vi "Table Select Section Cut to 1D Array.vi"(11 "Table Ref In":refnum<vi>) -> (1 "Cut Value":string[](array[string]), 3 "Table Ref Out":refnum<vi>)   [LabVIEW 2024]
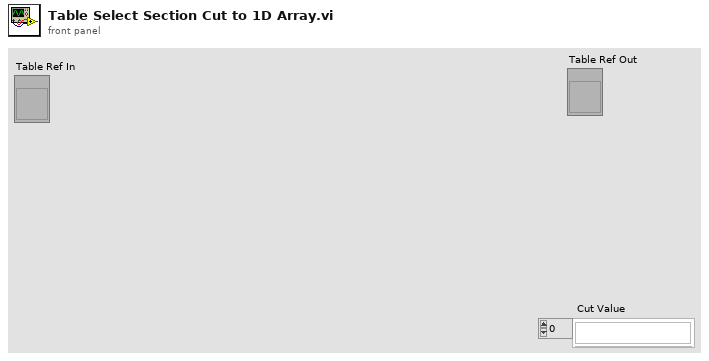
[diagram p1: front panel]
types:
  T1 = typedef "LVRowAndColumnTypeDef.ctl" = cluster{"Row":i32, "Column":i32}
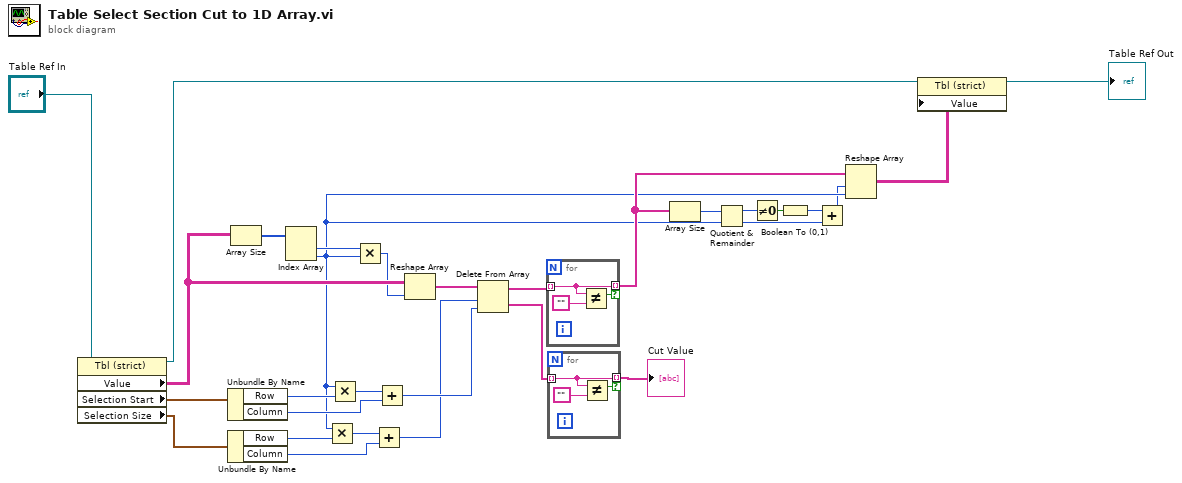
[diagram p0: block diagram]
diagram:
  n1 = property class="Tbl (strict)"(reference="Table Ref In") -> (reference out=w11:refnum<vi>, "Value"=w25:string[][], "Selection Start"=w29:T1, "Selection Size"=w28:T1)  [unwired: 1 in, 1 out]
  n2 = Unbundle By Name(w29) -> ("Row"=w23:i32, "Column"=w21:i32)
  n3 = Unbundle By Name(w28) -> ("Row"=w17:i32, "Column"=w16:i32)
  n4 = Array Size(array=w25) -> (size(s)=w27:i32[])
  n5 = Index Array(array=w27) -> (element #1=w26:i32, element #2=w7:i32)  [unwired: 2 in]
  n6 = Multiply(x=w7, y=w17) -> (x*y=w18:i32)
  n7 = Multiply(x=w7, y=w23) -> (x*y=w22:i32)
  n8 = Multiply(x=w26, y=w7) -> (x*y=w24:i32)
  n9 = Add(x=w18, y=w16) -> (x+y=w15:i32)
  n10 = Add(x=w22, y=w21) -> (x+y=w19:i32)
  n11 = Reshape Array(w25, w24) -> (w20:string[])
  n12 = Delete From Array(array=w20, length=w15, index=w19) -> (deleted portion=w13:string[], array with subset deleted=w14:string[])
  n13 = for {
    tunnel: [w31] -> w9 mode=indexing if=w32
    tunnel: w14 -> [w31] mode=indexing
    n14 = Not Equal?(x=w31, y="") -> (x != y?=w32:bool)
  }
  n15 = for {
    tunnel: [w34] -> w12 mode=indexing if=w35
    tunnel: w13 -> [w34] mode=indexing
    n16 = Not Equal?(x=w34, y="") -> (x != y?=w35:bool)
  }
  "Cut Value" <- w12
  n17 = Array Size(array=w9) -> (size(s)=w8:i32)
  n18 = Quotient & Remainder(x=w8, y=w7) -> (x-y*floor(x/y)=w6:i32, floor(x/y)=w2:i32)
  n19 = Not Equal To 0?(x=w6) -> (x != 0?=w4:bool)
  n20 = Boolean To (0,1)(Boolean=w4) -> (0, 1=w3:i16)
  n21 = Add(x=w3, y=w2) -> (x+y=w1:i32)
  n22 = Reshape Array(w9, w1, w7) -> (w5:string[][])
  n23 = property class="Tbl (strict)"(reference=w11, "Value"=w5) -> (reference out=→"Table Ref Out":refnum<vi>)  [unwired: 1 in, 1 out]
